vi "Configure Trigger Source.vi"(7 "Trigger External (T)":bool=TRUE, 8 "error in (no error)":errorcluster, 11 "VISA resource name":refnum<visa-resource-name>) -> (0 "error out":errorcluster, 3 "VISA resource name out":refnum<visa-resource-name>)   [LabVIEW 2020, in "QuPMXdriver.lvlib"]
doc: "Configures trigger source to external or internal."
uses:
  QuPMXdriver.lvlib
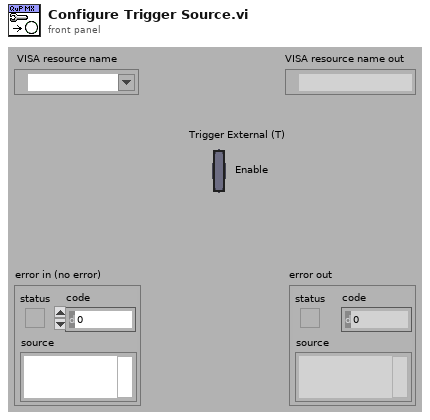
[diagram p1: front panel]
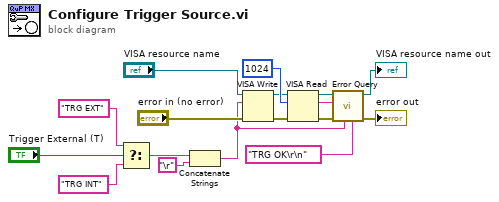
[diagram p0: block diagram]
diagram:
  n1 = Select(t="TRG EXT" ("write buffer"), s="Trigger External (T)", f="TRG INT" ("write buffer")) -> (s? t:f=w10:string)
  n2 = Concatenate Strings(w10, "\r") -> (w3:string)
  n3 = VISA Write(VISA resource name="VISA resource name", write buffer=w3, error in (no error)="error in (no error)") -> (VISA resource name out=w6:refnum<visa-resource-name>, error out=w1:errorcluster)  [unwired: 1 out]
  n4 = VISA Read(VISA resource name=w6, byte count=u32 1024, error in (no error)=w1) -> (VISA resource name out=w7:refnum<visa-resource-name>, read buffer=w4:string, error out=w5:errorcluster)  [unwired: 1 out]
  n5 = call "Error Query.vi"("Expected read buffer"="TRG OK\r\n" ("write buffer"), "Last command"=w3, "error in (no error)"=w5, "Read buffer"=w4, "VISA resource name"=w7) -> ("error out"=→"error out":errorcluster, "VISA resource name out"=→"VISA resource name out":refnum<visa-resource-name>)  [unwired: 5 in]
